vi "Add Transfer Group with Children.vi"(5 "buffer descriptor":T1={"buffer type"=enum."Engine", "plugin id"=-1, "group id"=-1, "transfer id"=-1, "offset"=0, "length"=-1}, 6 "ID":i32, 7 "Group Configuration":refnum<class "Group Configuration.lvclass">, 8 "error in (no error)":errorcluster, 9 "Plugin Decimation (1)":u64=1, 10 "parent tag":string, 11 "Application Data In":T3={"Item Tree Control"=refnum, "Top-Level VI"=refnum, "menu reference"=refnum, "queue"=refnum, "Stop Pointer"=refnum, "Buffer Variant"=variant, "server ID"=refnum, "framework tag"="", "Values"=refnum, "Hex"=refnum, "ASCII"=refnum, "lines visible"=0, "values padding"=0, "current buffer data"={"decimation"=0, "avg bandwidth"=0.0, "channels"=[], "byte order"=enum."little-endian", "buffer descriptor"={"buffer type"=enum."Engine", "plugin id"=0, "group id"=0, "transfer id"=0, "offset"=0, "length"=0}, "values channels"={"index"=0, "count"=0, "engine offset"=0}, "select start offset"=18446744073709551615, "select end offset"=0, "channel index"=-1}, "Framework Configuration"=refnum} {"current buffer data"."channels"."configuration"."string offset" format="%d bytes"; "current buffer data"."avg bandwidth" format="%.0g bytes"}) -> (0 "error out":errorcluster, 2 "average bandwidth":dbl format="%.0g bytes", 3 "Application Data In":T3={"Item Tree Control"=refnum, "Top-Level VI"=refnum, "menu reference"=refnum, "queue"=refnum, "Stop Pointer"=refnum, "Buffer Variant"=variant, "server ID"=refnum, "framework tag"="", "Values"=refnum, "Hex"=refnum, "ASCII"=refnum, "lines visible"=0, "values padding"=0, "current buffer data"={"decimation"=0, "avg bandwidth"=0.0, "channels"=[], "byte order"=enum."little-endian", "buffer descriptor"={"buffer type"=enum."Engine", "plugin id"=0, "group id"=0, "transfer id"=0, "offset"=0, "length"=0}, "values channels"={"index"=0, "count"=0, "engine offset"=0}, "select start offset"=18446744073709551615, "select end offset"=0, "channel index"=-1}, "Framework Configuration"=refnum} {"current buffer data"."channels"."configuration"."string offset" format="%d bytes"; "current buffer data"."avg bandwidth" format="%.0g bytes"})   [LabVIEW 2021, in "DSF Core.lvlib"]
uses:
  DSF Core.lvlib
  Main VI/Application Data.ctl
  <vilib>/NI/Memory Manager/Classes/Pointer/Pointer.lvclass
  Classes/Configuration/Core/Framework/Framework Configuration.lvclass
  Buffer Reader/Queue Data.ctl
  Buffer Reader/Buffer Data.ctl
  Classes/Configuration/Core/Transfer/Channel Configuration.ctl
  Typedefs/Core Channel Configuration.ctl
  Typedefs/DSF Data Type.ctl
  Typedefs/DSF Settings Info.ctl
  Typedefs/DSF Byte Order.ctl
  Classes/Thread/Data Server/DSF Buffer Subset Descriptor.ctl
  Typedefs/DSF Buffer Type.ctl
  Main VI/Values Channels.ctl
  Classes/Configuration/Core/Group/Group Configuration.lvclass
  ID to Tree Items/Tree Item Type.ctl
  Classes/Configuration/Core/Channel/Channel Configuration.lvclass
  Classes/Configuration/Core/Transfer/Transfer Configuration.lvclass
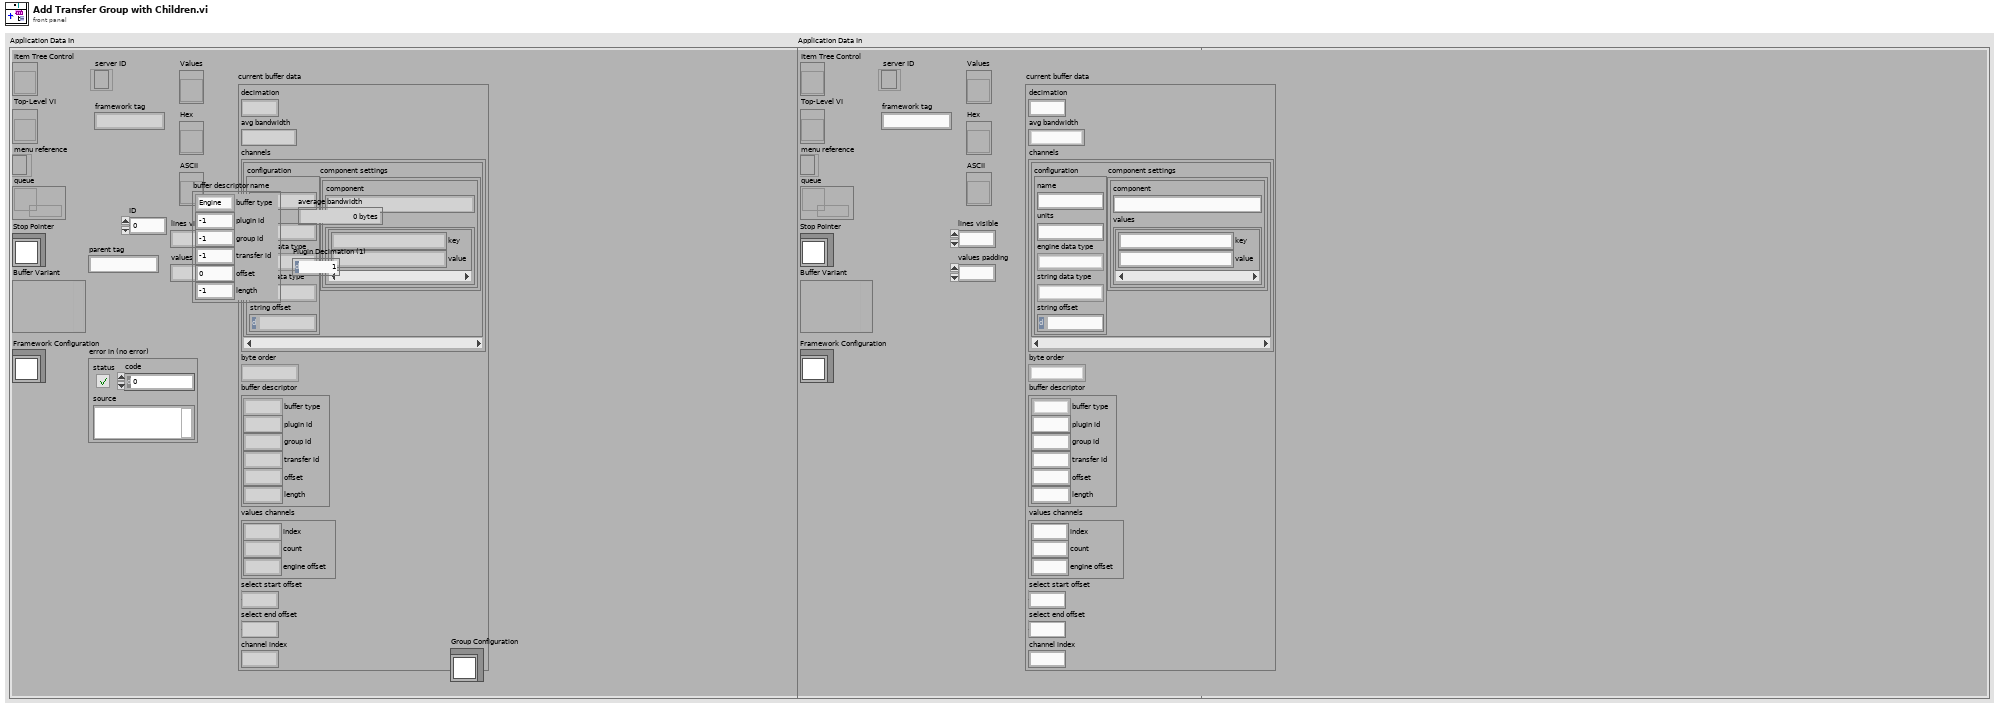
[diagram p1: front panel]
types:
  T1 = typedef "DSF Core.lvlib/DSF Buffer Subset Descriptor.ctl" = cluster{"buffer type":T2, "plugin id":i32, "group id":i32, "transfer id":i32, "offset":u64, "length":i64}
  T2 = typedef "DSF Core.lvlib/DSF Buffer Type.ctl" = enum16{"Engine", "String"}
  T3 = typedef "DSF Core.lvlib/Application Data.ctl" = cluster{"Item Tree Control":refnum<vi>, "Top-Level VI":refnum<vi>, "menu reference":refnum<k9>, "queue":refnum<queue>, "Stop Pointer":refnum<class "Pointer.lvclass">, "Buffer Variant":variant, "server ID":refnum<k5>, "framework tag":string, "Values":refnum<vi>, "Hex":refnum<vi>, "ASCII":refnum<vi>, "lines visible":i32, "values padding":i32, "current buffer data":T4, "Framework Configuration":refnum<class "Framework Configuration.lvclass">}
  T4 = typedef "DSF Core.lvlib/Buffer Data.ctl" = cluster{"decimation":u64, "avg bandwidth":dbl, "channels":T5[], "byte order":T9, "buffer descriptor":T1, "values channels":T10, "select start offset":u64, "select end offset":u64, "channel index":i32}
  T5 = typedef "DSF Core.lvlib/Transfer Configuration.lvclass/Channel Configuration.ctl" = cluster{"configuration":T6, "component settings":T8[]}
  T6 = typedef "DSF Core.lvlib/Channel Configuration.lvclass/Core Channel Configuration.ctl" = cluster{"name":string, "units":string, "engine data type":T7, "string data type":T7, "string offset":u64}
  T7 = typedef "DSF Core.lvlib/DSF Data Type.ctl" = enum8{"Bool", "SGL", "DBL", "I8", "I16", "I32", "I64", "U8", "U16", "U32", "U64"}
  T8 = typedef "DSF Core.lvlib/DSF Settings Info.ctl" = cluster{"component":string, "values":cluster{"key":string, "value":string}[]}
  T9 = typedef "DSF Core.lvlib/DSF Byte Order.ctl" = enum8{"big-endian", "little-endian"}
  T10 = typedef "DSF Core.lvlib/Values Channels.ctl" = cluster{"index":i32, "count":i32, "engine offset":u64}
  T11 = typedef "DSF Core.lvlib/Tree Item Type.ctl" = enum16{"Framework", "Plugin Group", "Plugin", "Group", "Transfer", "Buffer", "Channel"}
  T12 = typedef "DSF Core.lvlib/Group Configuration.lvclass/Core Group Configuration.ctl" = cluster{"name":string, "direction":T13, "cycle timing":T14, "timeout behavior":T15, "enable conversion":bool}
  T13 = typedef "DSF Core.lvlib/DSF Direction.ctl" = enum8{"Tx", "Rx"}
  T14 = typedef "DSF Core.lvlib/DSF Timing Info.ctl" = cluster{"priority":u64, "decimation":u64, "offset":u64}
  T15 = typedef "DSF Core.lvlib/DSF Timeout Behavior.ctl" = enum8{"Increment Late Count", "Throw Error"}
  T16 = typedef "DSF Core.lvlib/Tree Item.ctl" = cluster{"Left Cell String":string, "Child Text":string[], "Child Tag":string, "Glyph Index":i32}
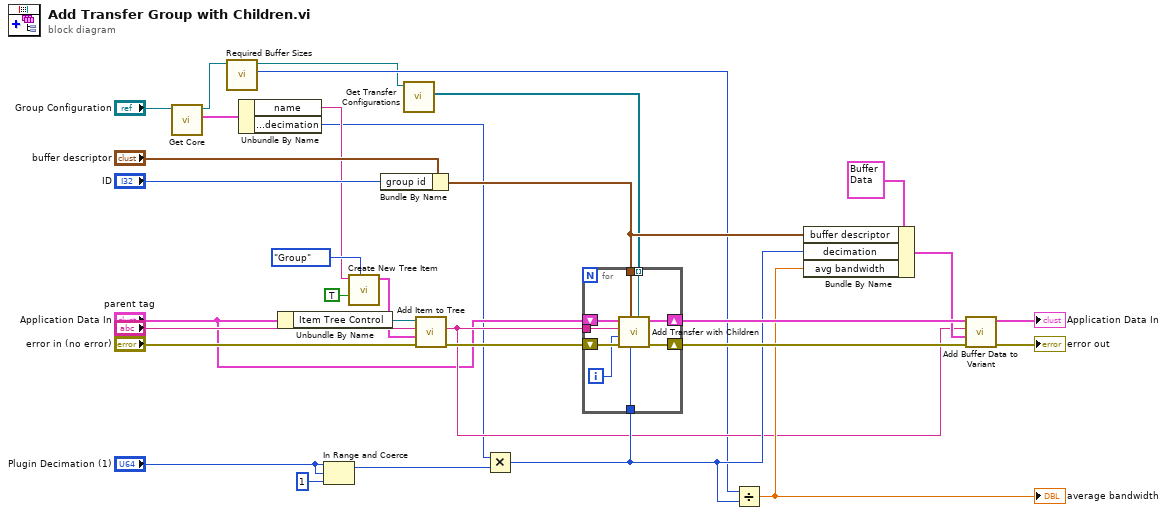
[diagram p0: block diagram]
diagram:
  n1 = call "Get Core.vi"("Group Configuration in"="Group Configuration") -> ("core"=w5:T12, "Group Configuration out"=w4:refnum<class "Group Configuration.lvclass">)  [unwired: 8 in, 1 out]
  n2 = call-dynamic "Required Buffer Sizes.vi"("Group Configuration in"=w4) -> ("engine size"=w3:u64, "Group Configuration out"=w2:refnum<class "Group Configuration.lvclass">)  [unwired: 7 in, 2 out]
  n3 = Unbundle By Name(w5) -> ("name"=w12:string, "cycle timing.decimation"=w7:u64)
  n4 = Unbundle By Name("Application Data In") -> ("Item Tree Control"=w27:refnum<vi>)
  n5 = In Range and Coerce(upper limit="Plugin Decimation (1)", x="Plugin Decimation (1)", lower limit=u64 1) -> (coerced(x)=w8:u64)  [unwired: 1 out]
  n6 = call "Create New Tree Item.vi"("Item Type"=Tree_Item_Type."Group", "found?"=TRUE, "Left Cell String"=w12) -> ("Item"=w28:T16)  [unwired: 7 in, 1 out]
  n7 = Bundle By Name(cluster="buffer descriptor", "group id"="ID") -> (w11:T1)
  n8 = call "Get Transfer Configurations.vi"("Group Configuration in"=w2) -> ("Transfer Configurations"=w1:refnum<class "Transfer Configuration.lvclass">[])  [unwired: 8 in, 2 out]
  n9 = call "Add Item to Tree.vi"("error in (no error)"="error in (no error)", "Item"=w28, "parent tag"="parent tag", "TreeControl in"=w27) -> ("error out"=w25:errorcluster, "new item tag"=w16:string)  [unwired: 5 in, 1 out]
  n10 = Multiply(x=w7, y=w8) -> (x*y=w17:u64)
  n11 = for {
    shift-right: [w38] -> w24
    shift-left: "Application Data In" -> [w40]
    shift-right: [w32] -> w23
    shift-left: w25 -> [w39]
    tunnel: w16 -> [w37]
    tunnel: w17 -> [w36]
    tunnel: w1 -> [w35] mode=indexing
    tunnel: w11 -> [w33]
    i -> [w34]
    n12 = call "Add Transfer with Children.vi"("Transfer Configuration"=w35, "Group Decimation (1)"=w36, "buffer descriptor"=w33, "error in (no error)"=w39, "Transfer ID"=w34, "parent tag"=w37, "Application Data In"=w40) -> ("error out"=w32:errorcluster, "Application Data Out"=w38:T3)  [unwired: 3 in]
  }
  n13 = Divide(x=w3, y=w17) -> (x/y=w19:dbl)
  "average bandwidth" <- w19
  n14 = Bundle By Name(cluster=T4 {"decimation"=0, "avg bandwidth"=0.0, "channels"=[], "byte order"=enum."big-endian", "buffer descriptor"={"buffer type"=enum."Engine", "plugin id"=0, "group id"=0, "transfer id"=0, "offset"=0, "length"=0}, "values channels"={"index"=0, "count"=0, "engine offset"=0}, "select start offset"=18446744073709551615, "select end offset"=0, "channel index"=-1} ("Buffer data"), "buffer descriptor"=w11, "decimation"=w17, "avg bandwidth"=w19) -> (w20:T4)
  n15 = call "Add Buffer Data to Variant.vi"("error in (no error)"=w23, "Buffer data"=w20, "tag"=w16, "Application Data In in"=w24) -> ("error out"=→"error out":errorcluster, "Application Data In out"=→"Application Data In":T3)  [unwired: 6 in]
